vi "高速脉冲占空比计算.vi"(11 "脉宽":dbl) -> (2 "占空比":dbl, 3 "周期":dbl)   [LabVIEW 2020, in "功能选择.xctl"]
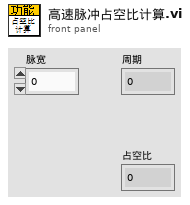
[diagram p1: front panel]
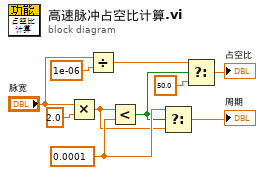
[diagram p0: block diagram]
diagram:
  w5 = 0.0001 ("y")
  n1 = Multiply(x="脉宽", y=2.0) -> (x*y=w2:dbl)
  n2 = Divide(x="脉宽", y=1e-06) -> (x/y=w7:dbl)
  n3 = Less?(x=w2, y=w5) -> (x < y?=w4:bool)
  n4 = Select(t=w5, s=w4, f=w2) -> (s? t:f=→"周期":dbl)
  n5 = Select(t=w7, s=w4, f=50.0) -> (s? t:f=→"占空比":dbl)
